vi "ReleaseMachine.vi"   [LabVIEW 2017]
uses:
  <vilib>/DAQmx/write.llb/DAQmx Write (Digital Bool 1Line 1Point).vi
  <vilib>/DAQmx/create/channels.llb/DAQmx Create Channel (DO-Digital Output).vi
  <vilib>/DAQmx/miscellaneous.llb/DAQmx Fill In Error Info.vi
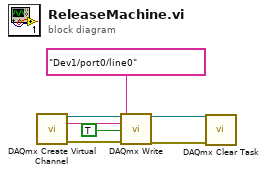
[diagram p0: block diagram]
diagram:
  n1 = call-poly <vilib>:"DAQmx Create Virtual Channel.vi"("lines"=tag "Dev1/port0/line0") -> ("task out"=w5:refnum<k21>, "error out"=w6:errorcluster)  [unwired: 13 in]
  n2 = call-poly <vilib>:"DAQmx Write.vi"("task/channels in"=w5, "data"=TRUE, "error in"=w6) -> ("task out"=w2:refnum<k21>, "error out"=w1:errorcluster)  [unwired: 10 in, 1 out]
  n3 = call <vilib>:"DAQmx Clear Task.vi"("task in"=w2, "error in"=w1) -> ()  [unwired: 13 in, 1 out]
